vi "Volume img-Load playback parameters.vi"(8 "error in (no error)":errorcluster) -> (0 "error out":errorcluster, 9 "AVI File Path":path=path "D:/Microscope data/10 Sep 2014/TimeLapse 10_09_2014 18-46-40 512x512/Experiment Header.ini")   [LabVIEW 2020]
uses:
  Functional Imaging Viewer/SubVIs/Experiment header interface/Typedefs/Header file sections.ctl
  Functional Imaging Viewer/SubVIs/Experiment header interface/Typedefs/Header file interface module functions enum.ctl
  Timelapse Viewer/Globals/gl_Time series viewer globals.vi
  Global Variables/General Globals.vi
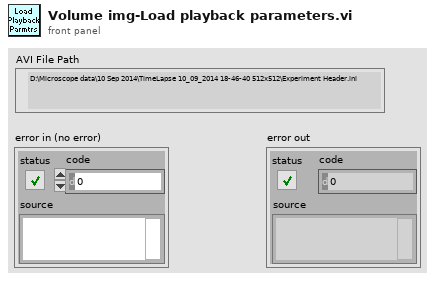
[diagram p1: front panel]
types:
  T1 = typedef "Time series viewer refs.ctl" = cluster{"This VI":refnum<vi>, "Image control":refnum<vi>, "AVI Mode ind":refnum<vi>, "Play":refnum<vi>, "Stop":refnum<vi>, "Back":refnum<vi>, "Scrollbar":refnum<vi>, "Video length info":refnum<vi>, "Expected speed values":refnum<vi>, "Intensity":refnum<vi>, "Path":refnum<vi>, "Selection sliders":refnum<vi>, "Speed Graph ref":refnum<vi>, "Frame rate set (fps)":refnum<vi>, "Number of rows to generate":refnum<vi>, "VL Image Array":refnum<vi>, "Image Scrollbar":refnum<vi>, "Channel to load":refnum<vi>, "Colour":refnum<vi>}
  T2 = typedef "Header file interface module functions enum.ctl" = enum16{"Load experiment header file", "Save experiment header file", "Clear stored values", "Read stored values", "Update specific value in memory", "Update values in memory"}
  T3 = typedef "Header file sections.ctl" = enum16{"ALL SECTIONS", "LOGIN", "GLOBAL PARAMETERS", "CALIBRATION DATA", "IMAGING MODES", "TIME SERIES", "MOTOR Z-STACK", "AOL Z-STACK", "FUNCTIONAL IMAGING", "VOLUME IMAGING", "MOVEMENT CORRECTION", "CALIBRATION", "STATISTICS", "BIOLOGY INFORMATION"}
  T4 = typedef "Header parameters cluster-ALL.ctl" = cluster{"LOGIN":T5, "GLOBAL PARAMETERS":T6, "IMAGING MODES":T8, "TIME SERIES":T9, "MOTOR Z-STACK ":T12, "AOL Z-STACK":T13, "FUNCTIONAL IMAGING":T14, "VOLUME IMAGING":T14, "MOVEMENT CORRECTION":T18, "CALIBRATION":T20, "STATISTICS":T21, "BIOLOGY INFORMATION":T22, "Calibration Data":T23}
  T5 = typedef "Header params -Login.ctl" = cluster{"User":string, "Profile":string, "Software Version":string, "Experiment Date Time":timestamp}
  T6 = typedef "Header params-Global Parameters.ctl" = cluster{"MicroscopeID":string, "Microscope Type":string, "Objective":string, "Field of View (um)":dbl, "Fill time (us)":dbl, "Experiment Type":T7, "Stimuli Trigger":bool, "Speed Logging":bool}
  T7 = typedef "Experiment Type.ctl" = enum16{"In vivo", "In vitro", "Testing", "Calibration", "Other"}
  T8 = typedef "Header params-Imaging Modes.ctl" = cluster{"Time Series":bool, "Motor Zstack":bool, "AOL Zstack":bool, "Functional Imaging":bool, "Volume Imaging":bool}
  T9 = typedef "Header params-Time Series.ctl" = cluster{"Basic Image meta data":T10, "AOL z":dbl}
  T10 = typedef "Header params-Basic image meta data.ctl" = cluster{"Wavelength (nm)":dbl, "# averaged frames":dbl, "laser power (%)":dbl, "Pockels":dbl, "pixel dwell time (us)":dbl, "pmt 1":dbl, "pmt 2":dbl, "back apperture":dbl, "zoom":dbl, "field of view":dbl, "Frame Size":T11, "AOL x centre":dbl, "AOL y centre":dbl, "Stage x position":dbl, "Stage y position":dbl, "Stage z position":dbl}
  T11 = typedef "Frame Size.ctl" = u16
  T12 = typedef "Header params-Motor Z-stack.ctl" = cluster{"Hdr Basic Image meta data":T10, "Z Start":dbl, "Z Stop":dbl, "No of Planes":i32, "Laser Power (%) at Z Start":dbl, "Laser Power (%) at Z Stop":dbl}
  T13 = typedef "Header params-AOL Z-stack.ctl" = cluster{"Hdr Basic Image meta data":T10, "Z Start":dbl, "Z Stop":dbl, "No of Planes":i32, "Laser Power (%) at Z Start":dbl, "Laser Power (%) at Z Stop":dbl}
  T14 = typedef "Header params-Functional Imaging.ctl" = cluster{"Functional Mode":T15, "Variable Length":bool, "Variable Resolution":bool, "Pockels Modulation":bool, "Stimuli Trigger":bool, "Cool down enabled":bool, "AOL Mode":T16, "Plane Mode":T17, "Miniscan Dwell time per pixel (us)":dbl, "poi dwell time":dbl, "Number of trials":dbl, "Number of cycles":dbl, "Number of pois":dbl, "Number of miniscans":dbl, "Number of pixels in miniscan":dbl, "Rectangle ROI length":dbl, "Rectangle ROI height":dbl, "Frame rate (fps)":dbl, "Acquisition Length":dbl, "video length (sec)":dbl, "Stimuli delay (sec)":dbl, "Cool down time (sec)":dbl, "Basic Image meta data":T10, "Z Start (um)":dbl, "Z Stop (um)":dbl}
  T15 = typedef "Functional Mode.ctl" = enum16{"Point", "Line", "Patch", "Plane", "Volume"}
  T16 = typedef "AOL modes.ctl" = enum16{"Raster", "Structural", "Pointing", "Mini Scan", "Alignment"}
  T17 = typedef "Plane Mode.ctl" = u16
  T18 = typedef "Header params-Movement correction.ctl" = cluster{"Movement Correction":bool, "Axial Reference":bool, "Reference Source":T19, "Full Frame Size":dbl, "Reference Field of View":dbl, "Reference Zoom":dbl, "Reference dwell time (us)":dbl, "Reference X Pixels":dbl, "Reference Y Pixels":dbl, "Number of Z lines":dbl, "Size of Z pixels":dbl, "Axial Pixels":dbl, "Ignore Z lines":dbl, "Reference Scan Cycles":dbl, "Reference Threshold XY":dbl, "Reference Threshold Z":dbl, "Reference Average XY":dbl, "Reference Average Z":dbl, "Proportional Scale":dbl, "Integral Scale":dbl, "Proportional Scale Z":dbl, "Integral Scale Z":dbl, "Diff Threshold":dbl, "Diff Threshold Z":dbl, "Sliding Average":bool, "Reference count reset enabled":bool, "Scan Interval (ms)":dbl, "Ref Plot Refresh Rate (ms)":dbl}
  T19 = typedef "Reference source.ctl" = enum16{"Green channel", "Red channel"}
  T20 = typedef "Header params-Calibration Setup.ctl" = cluster{"Pockels Calibration File":path, "Calibration_ini file":path, "Setup_ini file":path}
  T21 = typedef "Header params-statistics.ctl" = cluster{"Z-stack duration (sec)":dbl, "Number of acquired data-points":dbl, "Acquisition time (ms)":dbl, "Number of acquired frames":dbl, "Intertrial times":dbl[]}
  T22 = typedef "Biology Information.ctl" = cluster{"Animal Code or Name":string, "Animal DoB":string, "Animal Age":string, "Animal Sex":string, "Animal Weight":string, "Date of Injection":string, "Date of Implant":string, "Site of Injection":string, "Animal Ear Notch":string, "AAV constructs":string, "Genetic background":string, "Optical reporter":string, "Region of brain imaged":string, "Other \ncomments":string}
  T23 = typedef "Header params-calibration data.ctl" = cluster{"Objective Name":string, "Calibration Wavelength":dbl, "Sum X":dbl, "Sum Y":dbl, "Diff X":dbl, "Diff Y":dbl, "Distortion Correction":dbl, " Z norm to um Scaling":dbl, " X norm to um Scaling":dbl}
  T24 = typedef "AVI playback header info cluster.ctl" = cluster{"Frame Size":u32, "AOD fill time (us)":dbl, "Dwell time (us)":dbl, "Frame period (ms)":dbl, "Number of Miniscans":u16, "Number of Pixels in Miniscan":u16}
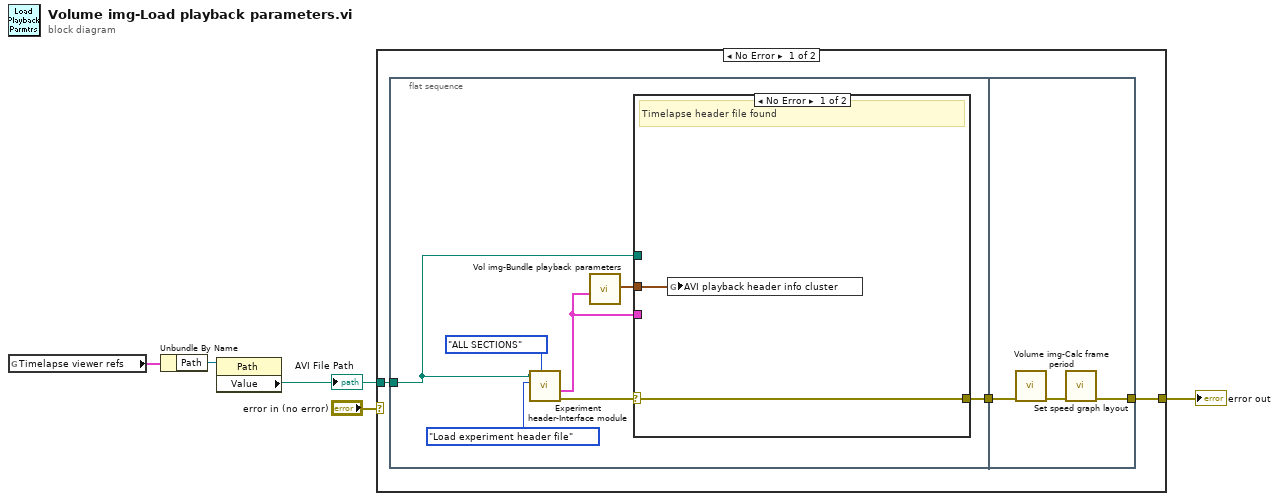
[diagram p0: block diagram]
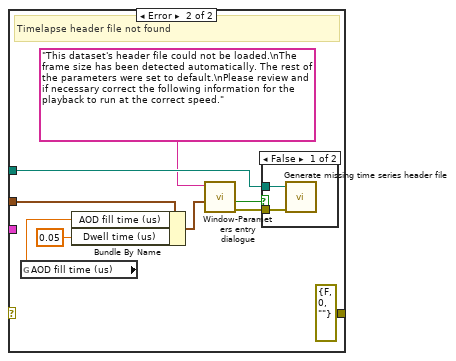
[diagram p2: hidden frame]
diagram:
  n1 = global read "gl_Time series viewer globals.vi" "Timelapse viewer refs"() -> (w3:T1)
  n2 = Unbundle By Name(w3) -> ("Path"=w2:refnum<vi>)
  n3 = property class="Path"(reference=w2) -> ("Value"=w1:path)  [unwired: 1 in, 2 out]
  "AVI File Path" <- w1
  n4 = case shown="No Error" "error in (no error)" {
    selector: "error in (no error)" -> [_ w32]
    tunnel: [w6 w32] -> w5
    tunnel: w1 -> [w8 _]
    frame No Error {
      n5 = flat-sequence {
        tunnel: w8 -> [w9]
        tunnel: [w12] -> w7
        tunnel: [w29] -> w6
        tunnel: w7 -> [w31]
        frame #0 {
          n6 = call "Experiment header-Interface module.vi"("Header file sections"=Header_file_sections."ALL SECTIONS", "Function"=Header_file_interface_module_functions_enum."Load experiment header file", "Experiment data folder path"=w9) -> ("error out"=w15:errorcluster, "All header parameters out"=w13:T4)  [unwired: 7 in]
          n7 = call "Vol img-Bundle playback parameters.vi"("All header parameters in"=w13) -> ("AVI playback header info cluster"=w14:T24)  [unwired: 10 in]
          n8 = case shown="No Error" w15 {
            selector: w15 -> [w16 _]
            tunnel: w13 -> [_ _]
            tunnel: w9 -> [_ w25]
            tunnel: w14 -> [w17 w21]
            tunnel: [w16 errorcluster {"status"=FALSE, "code"=0, "source"=""} ("error IO")] -> w12
            frame No Error {
              # "Timelapse header file found"
              n9 = global write "gl_Time series viewer globals.vi" "AVI playback header info cluster"(w17) -> ()
            }
            frame Error {
              # "Timelapse header file not found"
              n10 = global read "General Globals.vi" "AOD fill time (us)"() -> (w19:dbl)
              n11 = Bundle By Name(cluster=w21, "AOD fill time (us)"=w19, "Dwell time (us)"=0.05) -> (w22:T24)
              n12 = call "Window-Parameters entry dialogue.vi"("AVI playback header info cluster"=w22, "Message"="This dataset's header file could not be loaded.\nThe frame size has been detected automatically. The rest of the parameters were set to default.\nPlease review and if necessary correct the following information for the playback to run at the correct speed.") -> ("error out"=w26:errorcluster, "Cancelled"=w23:bool)  [unwired: 8 in]
              n13 = case shown="False" w23 {
                tunnel: w26 -> [w28 _]
                tunnel: w25 -> [w27 _]
                frame False {
                  n14 = call "Generate missing time series header file.vi"("error in (no error)"=w28, "Timelapse data folder path"=w27) -> ()  [unwired: 10 in]
                }
                frame True {
                }
              }
            }
          }
        }
        frame #1 {
          n15 = call "Volume img-Calc frame period.vi"("error in (no error)"=w31) -> ("error out"=w30:errorcluster)  [unwired: 10 in]
          n16 = call "Set speed graph layout.vi"("error in (no error)"=w30) -> ("error out"=w29:errorcluster)  [unwired: 10 in]
        }
      }
    }
    frame Error {
    }
  }
  "error out" <- w5
